vi "Home(HOM).vi"(2 "AXIS":u16(ring) items=["X", "Y", "X&Y"], 3 "baud rate (9600)":u32=115200 caption="보 전송속도(9600)", 4 "Port":refnum<visa-resource-name>="COM4" caption="VISA 리소스 이름") -> (0 "Error Out":errorcluster caption="에러 출력", 1 "VISA out":refnum<visa-resource-name>)   [LabVIEW 2010]
uses:
  <vilib>/Instr/_visa.llb/VISA Flush IO Buffer Mask.ctl
  <vilib>/Instr/_visa.llb/VISA Configure Serial Port (Instr).vi
panel:
  out "Commend Count":u32
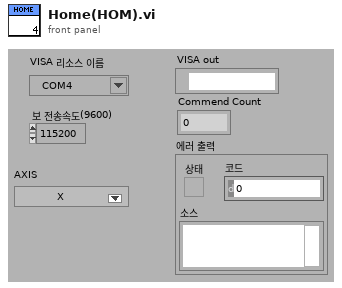
[diagram p1: front panel]
types:
  T1 = typedef "VISA Flush IO Buffer Mask.ctl" = u16
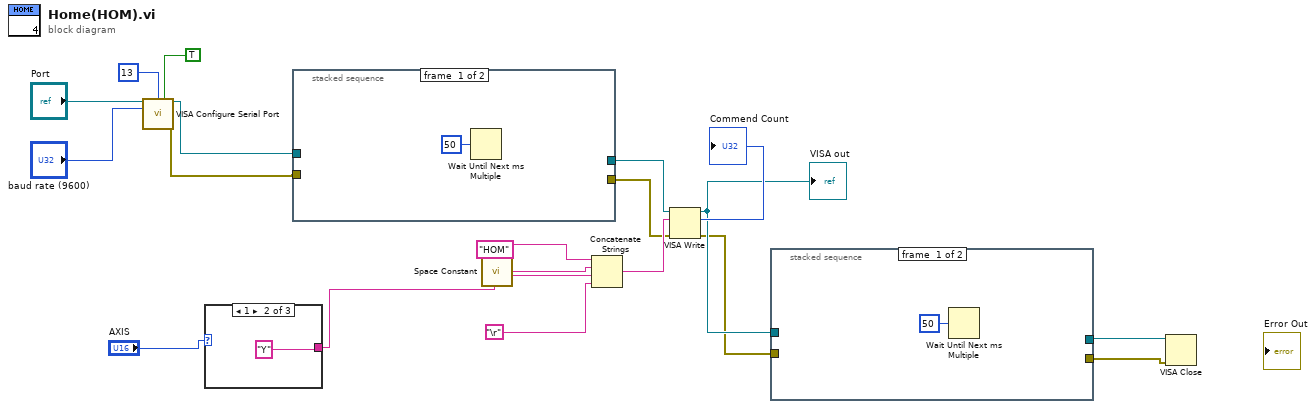
[diagram p0: block diagram]
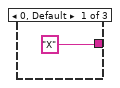
[diagram p2: hidden frame]
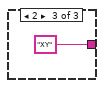
[diagram p3: hidden frame]
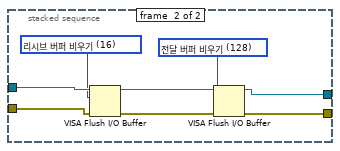
[diagram p4: hidden frame]
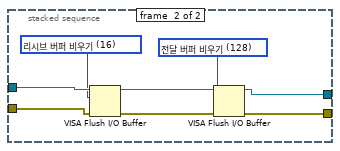
[diagram p5: hidden frame]
diagram:
  n1 = call-poly "VISA Configure Serial Port"("VISA resource name"="Port", "termination char\n(0xA = '\\n' = LF)"=i16 13 ("termination char\n(0xA = '\\n' = LF)"), "Enable Termination\nChar (T)"=TRUE ("Enable Termination\nChar (T)"), "baud rate (9600)"="baud rate (9600)") -> ("VISA resource name out"=w4:refnum<visa-resource-name>, "error out"=w3:errorcluster)  [unwired: 10 in]
  n2 = case shown="1" "AXIS" {
    tunnel: ["X" "Y" "XY"] -> w1
    frame 0, Default {
    }
    frame 1 {
    }
    frame 2 {
    }
  }
  n3 = stacked-sequence {
    tunnel: w4 -> [_ w31]
    tunnel: w3 -> [_ w30]
    tunnel: [_ w26] -> w10
    tunnel: [_ w25] -> w9
    frame #0 {
      n4 = Wait Until Next ms Multiple(millisecond multiple=u32 50 ("ms 배수")) -> ()  [unwired: 1 out]
    }
    frame #1 {
      w24 = T1 128 items=["리시브 버퍼 비우기"=16, "전달 버퍼 디바이스에 쓰기"=32, "리시브 버퍼 비우기(I/O 없음)"=64, "전달 버퍼 비우기"=128] ("Mask")
      w29 = T1 16 items=["리시브 버퍼 비우기"=16, "전달 버퍼 디바이스에 쓰기"=32, "리시브 버퍼 비우기(I/O 없음)"=64, "전달 버퍼 비우기"=128] ("Mask")
      n5 = VISA Flush I/O Buffer(VISA resource name=w31, mask (16)=w29, error in (no error)=w30) -> (VISA resource name out=w28:refnum<visa-resource-name>, error out=w27:errorcluster)
      n6 = VISA Flush I/O Buffer(VISA resource name=w28, mask (16)=w24, error in (no error)=w27) -> (VISA resource name out=w26:refnum<visa-resource-name>, error out=w25:errorcluster)
    }
  }
  n7 = call <vilib>:"Space Constant.vi"() -> ("String"=w18:string)
  n8 = Concatenate Strings("HOM", w18, w1, "\r") -> (w16:string)
  n9 = VISA Write(VISA resource name=w10, write buffer=w16, error in (no error)=w9) -> (VISA resource name out=w12:refnum<visa-resource-name>, return count=→"Commend Count":u32, error out=w11:errorcluster)
  "VISA out" <- w12
  n10 = stacked-sequence {
    tunnel: w12 -> [_ w40]
    tunnel: w11 -> [_ w39]
    tunnel: [_ w35] -> w14
    tunnel: [_ w34] -> w13
    frame #0 {
      n11 = Wait Until Next ms Multiple(millisecond multiple=u32 50 ("ms 배수")) -> ()  [unwired: 1 out]
    }
    frame #1 {
      w33 = T1 128 items=["리시브 버퍼 비우기"=16, "전달 버퍼 디바이스에 쓰기"=32, "리시브 버퍼 비우기(I/O 없음)"=64, "전달 버퍼 비우기"=128] ("Mask")
      w38 = T1 16 items=["리시브 버퍼 비우기"=16, "전달 버퍼 디바이스에 쓰기"=32, "리시브 버퍼 비우기(I/O 없음)"=64, "전달 버퍼 비우기"=128] ("Mask")
      n12 = VISA Flush I/O Buffer(VISA resource name=w40, mask (16)=w38, error in (no error)=w39) -> (VISA resource name out=w37:refnum<visa-resource-name>, error out=w36:errorcluster)
      n13 = VISA Flush I/O Buffer(VISA resource name=w37, mask (16)=w33, error in (no error)=w36) -> (VISA resource name out=w35:refnum<visa-resource-name>, error out=w34:errorcluster)
    }
  }
  n14 = VISA Close(VISA resource name=w14, error in (no error)=w13) -> ()  [unwired: 1 out]
